vi "Map Input to Output.vi"(5 "output Range":T1 {"Low" format="%#.8f"; "High" format="%#.8f"}, 7 "Input Range":T1 {"Low" format="%#.8f"; "High" format="%#.8f"}, 11 "Input":dbl) -> (3 "output":dbl)   [LabVIEW 2020]
uses:
  Shared Code/TypeDefs/Cluster_High-Low.ctl
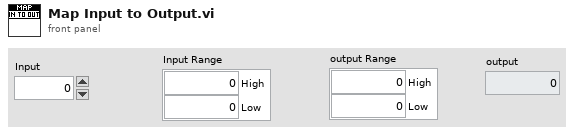
[diagram p1: front panel]
types:
  T1 = typedef "Cluster_High-Low.ctl" = cluster{"High":dbl, "Low":dbl}
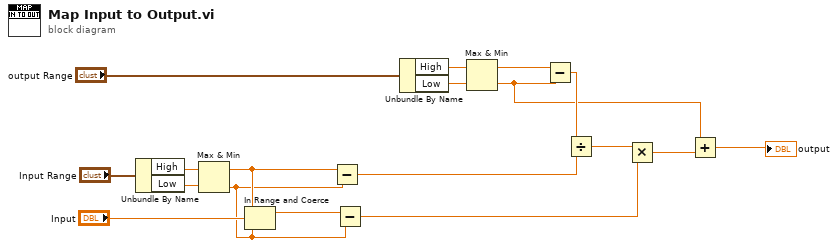
[diagram p0: block diagram]
diagram:
  n1 = Unbundle By Name("Input Range") -> ("High"=w16:dbl, "Low"=w15:dbl)
  n2 = Max & Min(x=w16, y=w15) -> (max(x,y)=w14:dbl, min(x,y)=w4:dbl)
  n3 = In Range and Coerce(upper limit=w14, x="Input", lower limit=w4) -> (coerced(x)=w5:dbl)  [unwired: 1 out]
  n4 = Subtract(x=w14, y=w4) -> (x-y=w8:dbl)
  n5 = Subtract(x=w5, y=w4) -> (x-y=w2:dbl)
  n6 = Unbundle By Name("output Range") -> ("High"=w11:dbl, "Low"=w12:dbl)
  n7 = Max & Min(x=w11, y=w12) -> (max(x,y)=w10:dbl, min(x,y)=w7:dbl)
  n8 = Subtract(x=w10, y=w7) -> (x-y=w9:dbl)
  n9 = Divide(x=w9, y=w8) -> (x/y=w3:dbl)
  n10 = Multiply(x=w3, y=w2) -> (x*y=w1:dbl)
  n11 = Add(x=w7, y=w1) -> (x+y=→"output":dbl)
